vi "FocalSpot.vi"(7 "Racine chemin de sauvegarde":path=path "Z:/Data Gas Experiments/Spring2019/Taches Focales") -> ()   [LabVIEW 2014]
uses:
  <vilib>/addons/PixeLINK/Low Level Functions/ACQUISITION.llb/TDPU-Acquisition-StreamState.ctl
  <vilib>/addons/PixeLINK/Low Level Functions/CAMERA_FEATURES.llb/TDPU-CameraFeatures-FeatureIds.ctl
  <vilib>/addons/PixeLINK/Low Level Functions/CAMERA_FEATURES.llb/TDPU-CameraFeatures-FeatureFlags.ctl
  <vilib>/Analysis/5stat.llb/RMS (DBL).vi
  <vilib>/Analysis/baseanly.llb/Mean (DBL).vi
  <vilib>/Analysis/NI_AALPro.lvlib
  <vilib>/Analysis/NI_AALBase.lvlib
  <vilib>/Utility/file.llb/Write To Spreadsheet File (I64).vi
panel:
  in  "Zoom":bool
  out "rms value":dbl format="%0.2f"
  out "mean":dbl format="%0.2f"
  out "BKG OK":bool
  out "ROI OK":bool
  out "Background":dbl[][](graph)
  in  "Select Background":bool
  out "ROI":dbl[][](graph)
  in  "Select ROI":bool
  in  "Stop Acquisition":bool
  in  "Refresh Exposure":bool
  in  "Transmission":dbl=0.5
  out "Intensity (measured)\nx10^18 W/cm²":dbl=2.0
  out "Div":dbl
  in  "Automatic\nfolder naming":bool=TRUE
  in  "Imager":u32(ring) items=["Low Res Side View"=957000275, "Focal Spot"=953000197, "High Res Side View"=95300230]
  out "?":dbl[][](graph)
  out "?":dbl[][](graph)
  in  "Background  substraction":bool
  out "Intensity (gaussian)\nx10^18 W/cm²":dbl=2.0
  out "Peak power (TW)":dbl=2.0
  out "FWHM y (µm)":dbl=2.0
  out "FWHM x (µm)":dbl=2.0
  in  "Duration FWHM (fs)":dbl=4.5
  in  "Pulse Energy (mJ)":dbl=5.0
  in  "Calibration µm/px":dbl=0.135
  out "Error OUT 2":errorcluster
  out "Error OUT":errorcluster
  in  "Overwrite?":bool
  in  "Snap current Data":bool
  in  "Save Data":bool
  out "Warning":bool
  out "Message":string
  in  "Indice":u32
  in  "Nom du fichier":string="TacheFocale"
  in  "Mode de Sauvegarde":u16(ring)=1 items=["Manuel", "Automatique"]
  out "Focal Spot":dbl[][](graph)
  out "Waiting for Trigger":bool
  in  "Continuous Grab":bool
  in  "Snap Next frame":bool
  out "Camera Handle":u32
  in  "Trigger Type":enum16{"Free Running", "Software", "Hardware"}(ring)
  in  "Trigger Polarity":enum16{"Positive", "Negative"}(ring)
  in  "Refresh Trigger":bool
  in  "Exposure Time":dbl(slide) min=0.0 max=0.0 scale=0.01..10.0
  in  "stop":bool
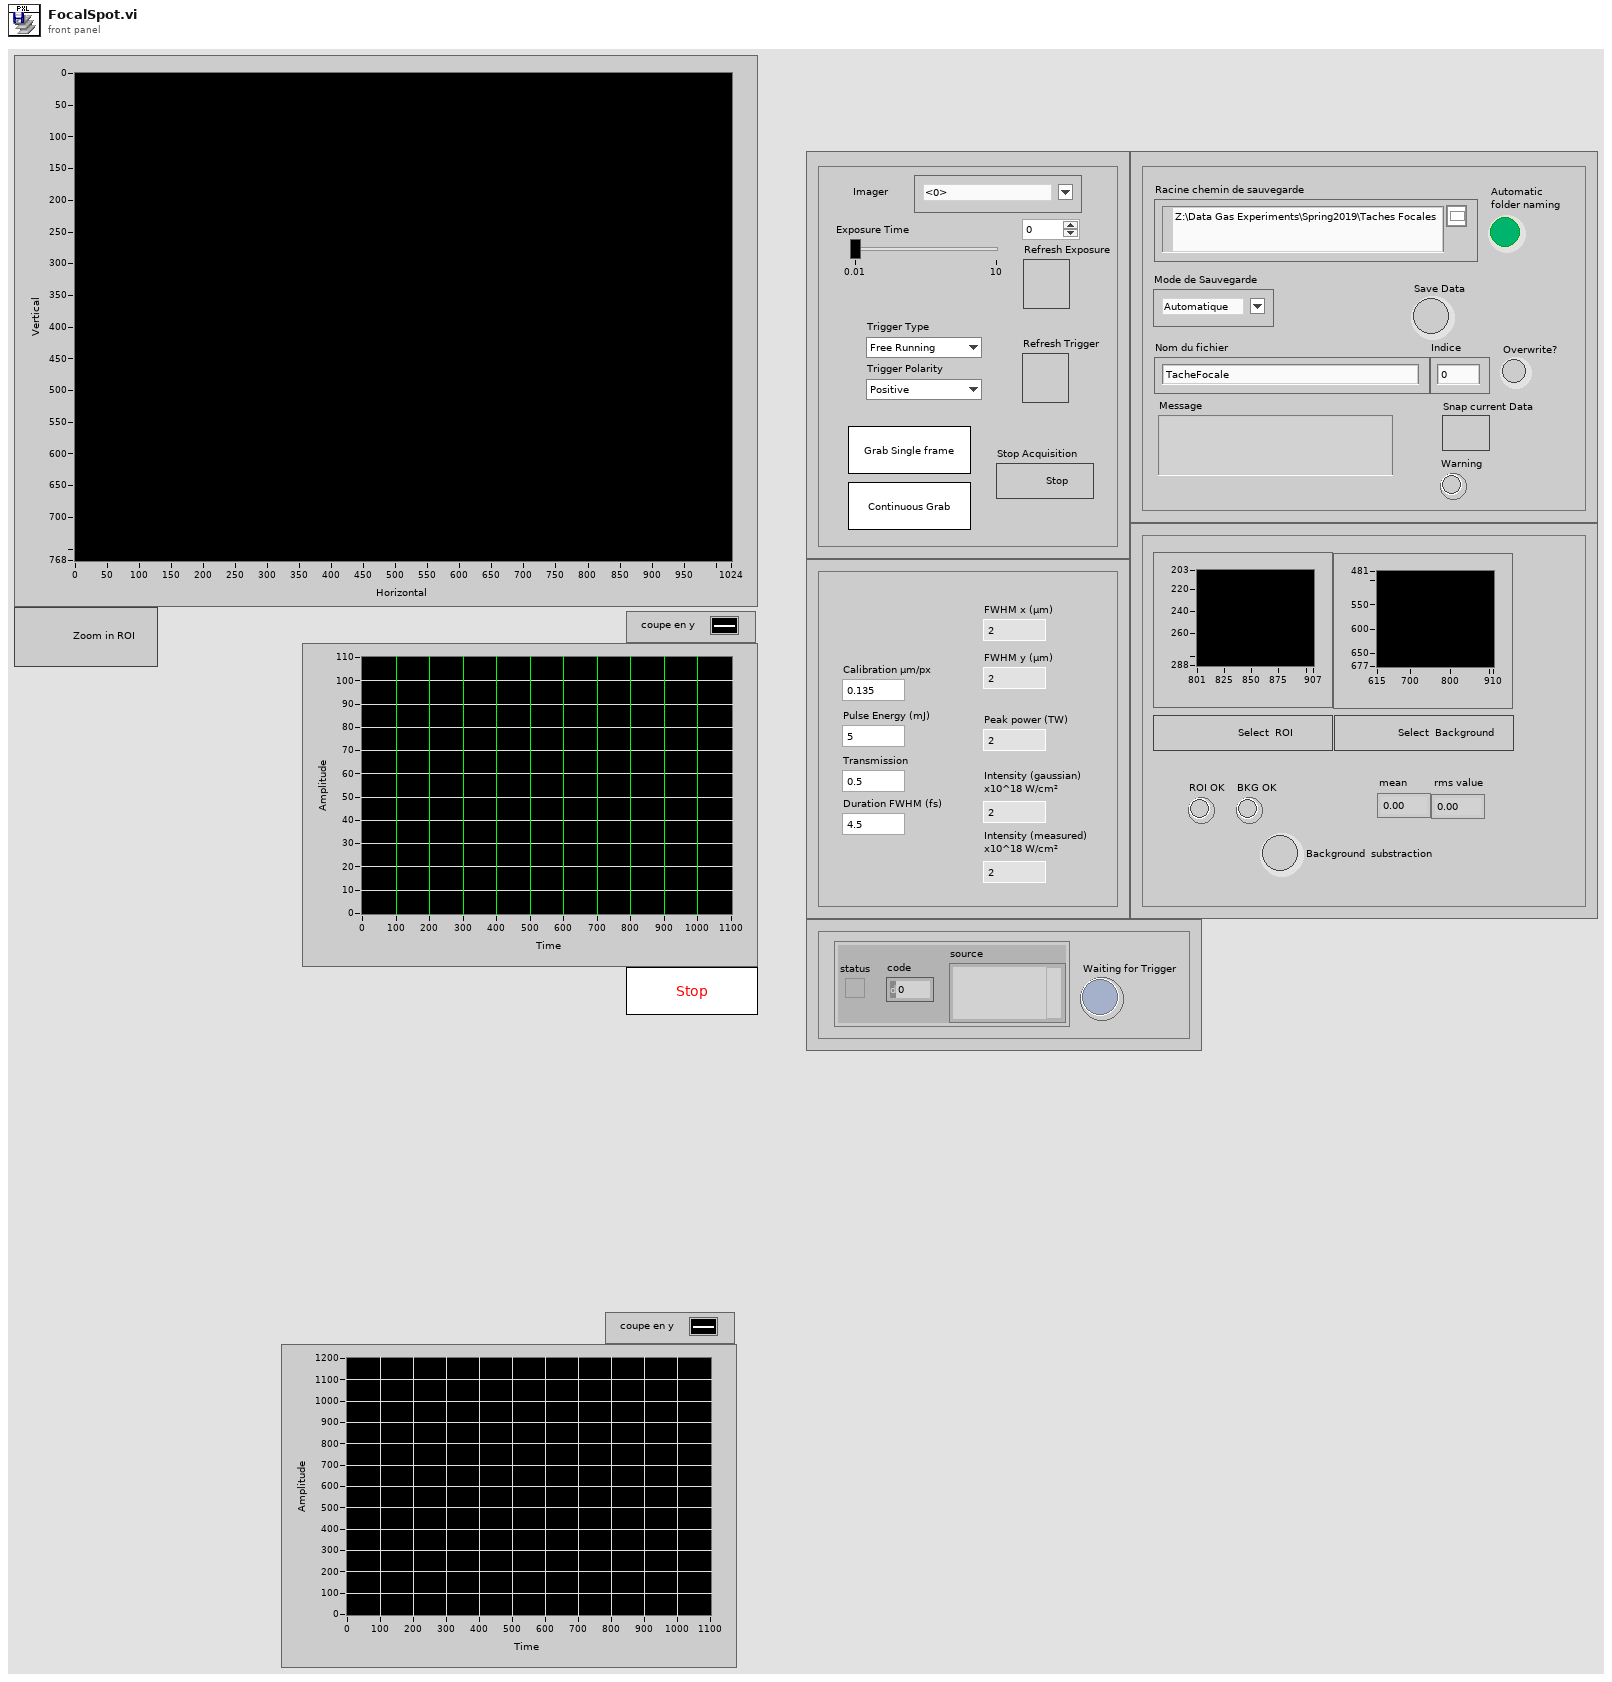
[diagram p1: front panel]
types:
  T1 = typedef "LVStringsAndValuesArrayTypeDef_U32.ctl" = cluster{"String":string, "Value":u32}[]
  T2 = typedef "TDPU-CameraFeatures-FeatureFlags.ctl" = u32
  T3 = typedef "TDPU-CameraFeatures-FeatureIds.ctl" = u32
  T4 = typedef "TDPU-Acquisition-StreamState.ctl" = u32
  T5 = typedef "TDPU-Identification-Camera_Info.ctl" = cluster{"VendorName":string, "ModelName":string, "Description":string, "SerialNumber":string, "FirmwareVersion":string, "FPGAVersion":string, "CameraName":string}
  T6 = typedef "TDPU-Acquisition-Frame_Desc.ctl" = cluster{"uSize":u32, "fFrameTime":dbl, "uFrameNumber":u32, "Brightness":cluster{"fValue":dbl}, "AutoExposure":cluster{"fValue":dbl}, "Sharpness":cluster{"fValue":dbl}, "WhiteBalance":cluster{"fValue":dbl}, "Hue":cluster{"fValue":dbl}, "Saturation":cluster{"fValue":dbl}, "Gamma":cluster{"fValue":dbl}, "Shutter":cluster{"fValue":dbl}, "Gain":cluster{"fValue":dbl}, "Iris":cluster{"fValue":dbl}, "Focus":cluster{"fValue":dbl}, "Temperature":cluster{"fValue":dbl}, "Trigger":cluster{"fMode":dbl, "fType":dbl, "fPolarity":dbl, "fDelay":dbl, "fParameter":dbl}, "Zoom":cluster{"fValue":dbl}, "Pan":cluster{"fValue":dbl}, "Tilt":cluster{"fValue":dbl}, "OpticalFilter":cluster{"fValue":dbl}, "GPIO":cluster{"fMode":dbl[], "fPolarity":dbl[], "fParameter1":dbl[], "fParameter2":dbl[], "fParameter3":dbl[]}, "FrameRate":cluster{"fValue":dbl}, "ROI":cluster{"fLeft":dbl, "fTop":dbl, "fWidth":dbl, "fHeight":dbl}, "Flip":cluster{"fHorizontal":dbl, "fVertical":dbl}, "PixelAddressingValue":cluster{"fValue":dbl}, "PixelFormat":cluster{"fValue":dbl}, "ExtendedShutter":cluster{"fKneePoint":dbl[]}, "AutoROI":cluster{"fLeft":dbl, "fTop":dbl, "fWidth":dbl, "fHeight":dbl}, "WhiteShading":cluster{"fRedGain":dbl, "fGreenGain":dbl, "fBlueGain":dbl}, "Rotate":cluster{"fValue":dbl}, "PixelAddressingMode":cluster{"fValue":dbl}}
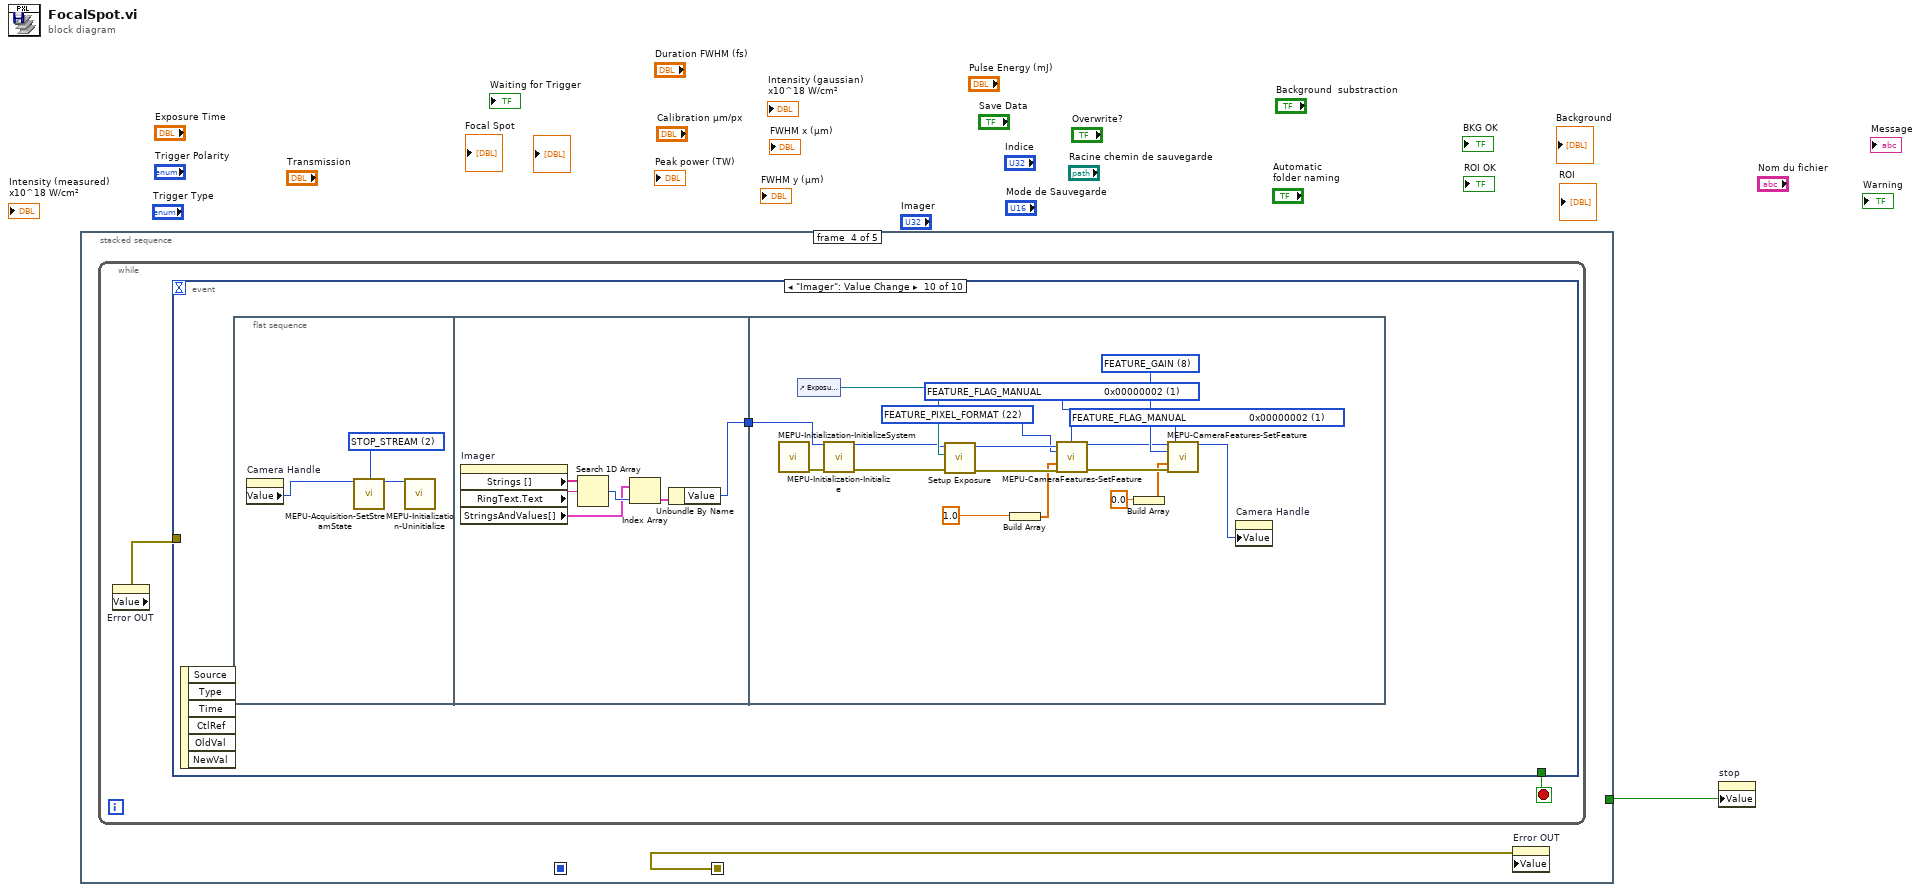
[diagram p0: block diagram]
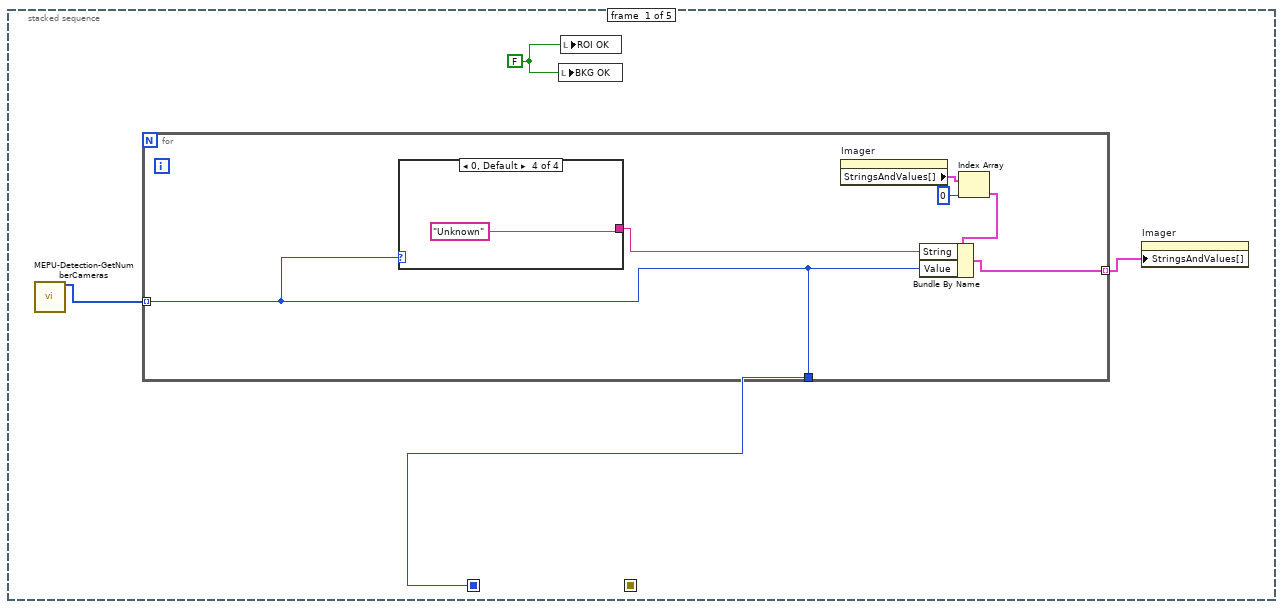
[diagram p2: hidden frame]
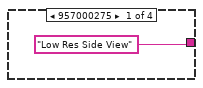
[diagram p3: hidden frame]
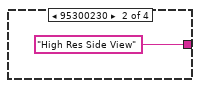
[diagram p4: hidden frame]
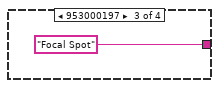
[diagram p5: hidden frame]
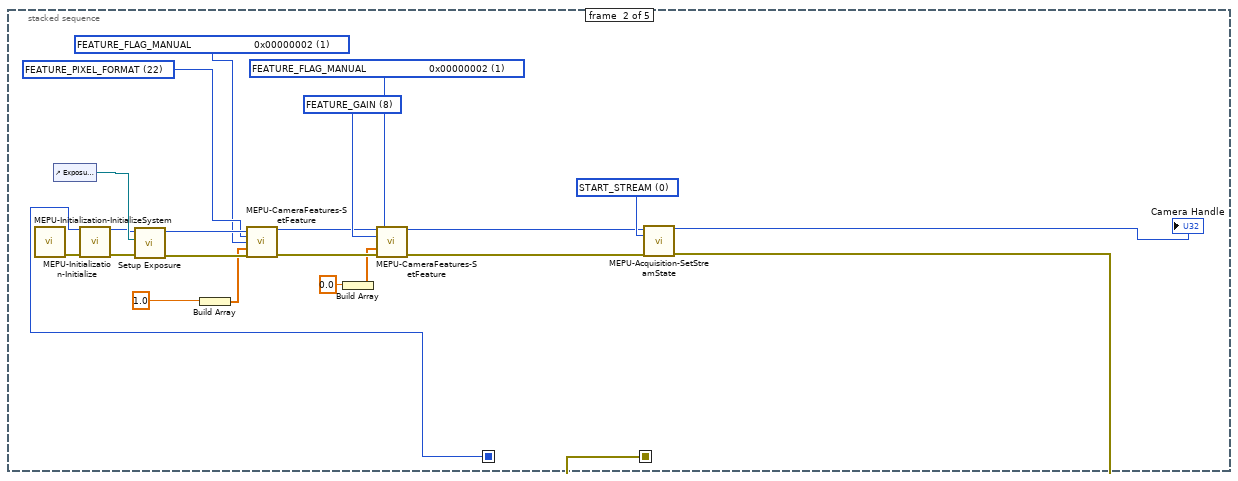
[diagram p6: hidden frame]
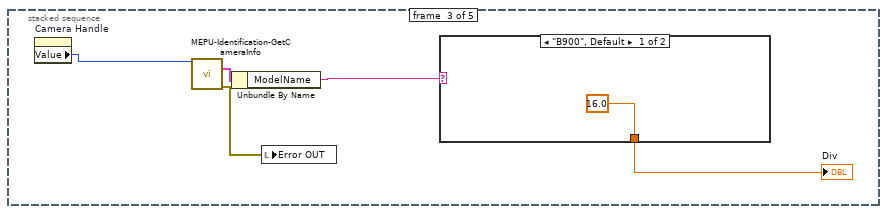
[diagram p7: hidden frame]
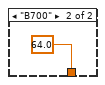
[diagram p8: hidden frame]
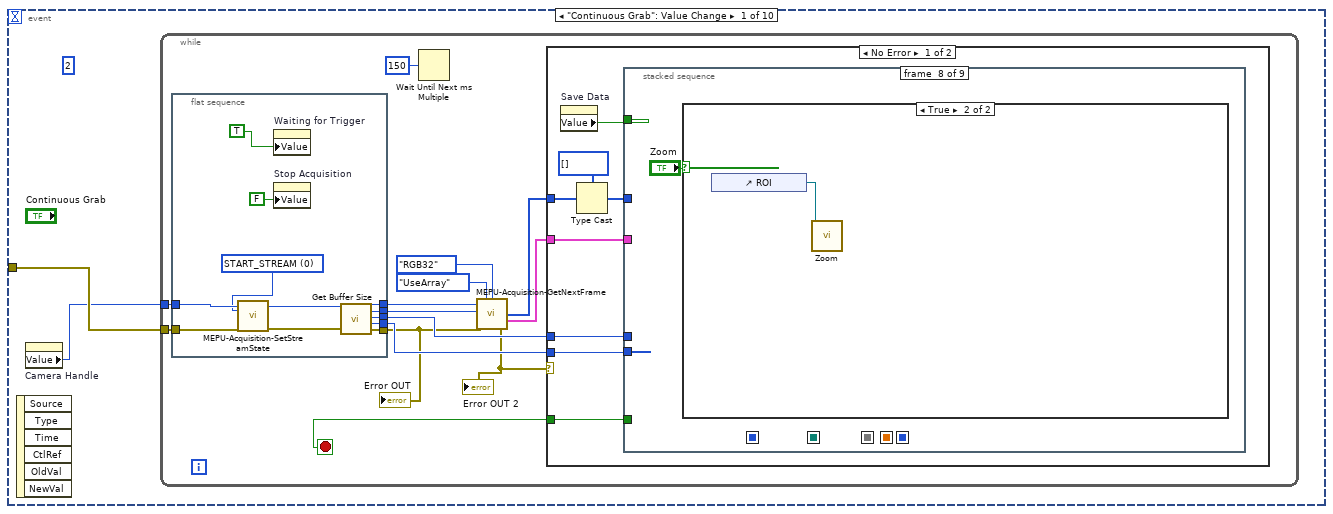
[diagram p9: hidden frame]
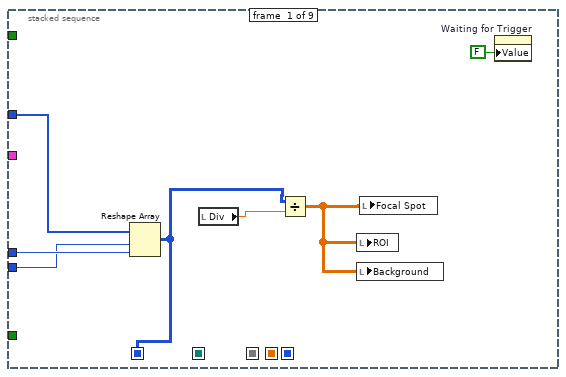
[diagram p10: hidden frame]
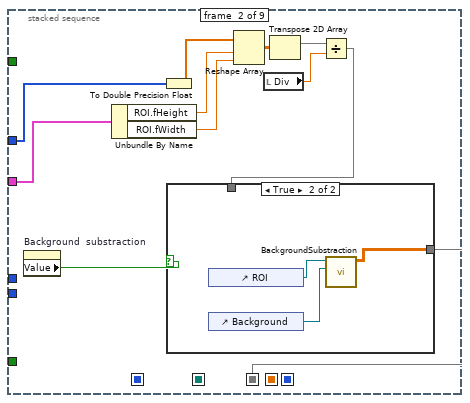
[diagram p11: hidden frame]
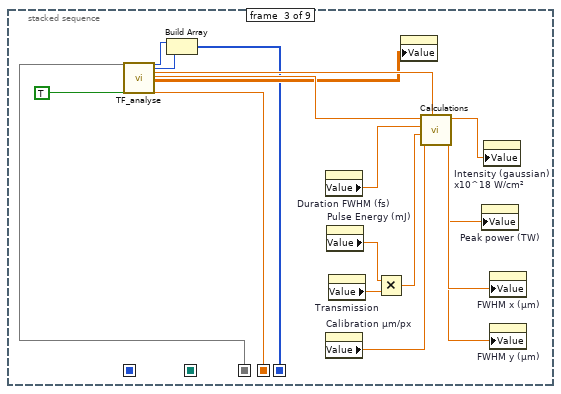
[diagram p13: hidden frame]
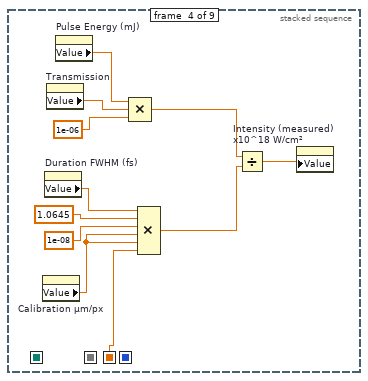
[diagram p14: hidden frame]
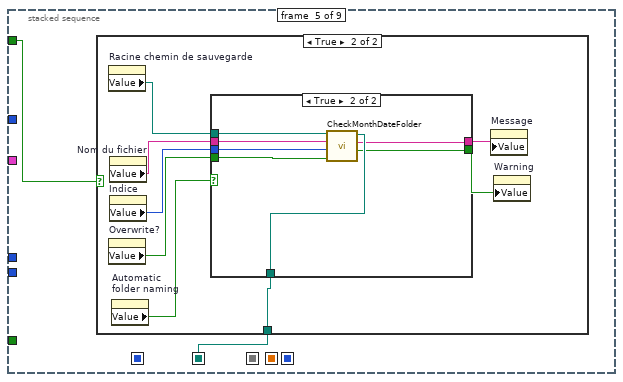
[diagram p15: hidden frame]
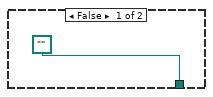
[diagram p16: hidden frame]
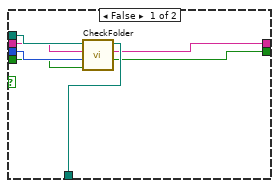
[diagram p17: hidden frame]
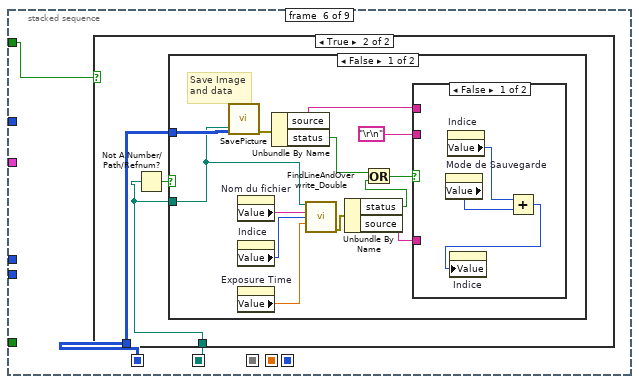
[diagram p18: hidden frame]
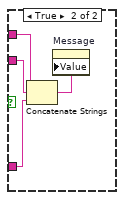
[diagram p20: hidden frame]
diagram:
  n1 = stacked-sequence {
    seq-local: [_ w26 _ _ _] -> [_ _ _ w45 _]
    seq-local: [w3 _ _ _ _] -> [_ w16 _ _ _]
    tunnel: [_ _ _ _ TRUE] -> w1
    frame #0 {
      w2 = FALSE
      n2 = call <vilib>:"MEPU-Detection-GetNumberCameras.vi"() -> ("LV_SerialNumbers OUT"=w5:u32[])  [unwired: 13 in, 2 out]
      n3 = for {
        tunnel: w5 -> [w7] mode=indexing
        tunnel: [w8] -> w4 mode=indexing
        tunnel: [w7] -> w3
        n4 = case shown="0, Default" w7 {
          tunnel: ["Low Res Side View" "High Res Side View" "Focal Spot" "Unknown"] -> w6
          frame 957000275 {
          }
          frame 95300230 {
          }
          frame 953000197 {
          }
          frame 0, Default {
          }
        }
        n5 = property on="Imager" class="Ring (strict)"() -> ("StringsAndValues[]"=w11:T1)  [unwired: 2 in, 2 out]
        n6 = Index Array(array=w11, index=0) -> (element=w9:cluster{"String":string, "Value":u32})
        n7 = Bundle By Name(cluster=w9, "String"=w6, "Value"=w7) -> (w8:cluster{"String":string, "Value":u32})
      }
      n8 = local write "BKG OK"(w2) -> ()
      n9 = local write "ROI OK"(w2) -> ()
      n10 = property on="Imager" class="Ring (strict)"("StringsAndValues[]"=w4) -> ()  [unwired: 2 in, 2 out]
    }
    frame #1 {
      w21 = T2 1 items=["FEATURE_FLAG_PRESENCE                 0x00000001", "FEATURE_FLAG_MANUAL                     0x00000002", "FEATURE_FLAG_AUTO                         0x00000004", "FEATURE_FLAG_ONEPUSH                   0x00000008", "FEATURE_FLAG_OFF                            0x00000010", "FEATURE_FLAG_DESC_SUPPORTED    0x00000020", "FEATURE_FLAG_READ_ONLY               0x00000040"] ("uFlags IN")
      w20 = T3 8 items=["FEATURE_BRIGHTNESS", "FEATURE_EXPOSURE", "FEATURE_SHARPNESS", "FEATURE_WHITE_BAL", "FEATURE_HUE", "FEATURE_SATURATION", "FEATURE_GAMMA", "FEATURE_SHUTTER", "FEATURE_GAIN", "FEATURE_IRIS", "FEATURE_FOCUS", "FEATURE_TEMPERATURE", "FEATURE_TRIGGER", "FEATURE_ZOOM", "FEATURE_PAN", "FEATURE_TILT", "FEATURE_OPT_FILTER", "FEATURE_GPIO", "FEATURE_FRAME_RATE", "FEATURE_ROI", "FEATURE_FLIP", "FEATURE_PIXEL_ADDRESSING", "FEATURE_PIXEL_FORMAT", "FEATURE_EXTENDED_SHUTTER", "FEATURE_AUTO_ROI", "FEATURE_LOOKUP_TABLE", "FEATURE_MEMORY_CHANNEL", "FEATURE_WHITE_SHADING", "FEATURE_ROTATE", "FEATURE_IMAGER_CLK_DIVISOR", "FEATURE_TRIG_WITH_CNTRLD_LIGHT", "FEATURE_MAX_PIXEL_SIZE"] ("uFeatureId IN")
      w29 = T2 1 items=["FEATURE_FLAG_PRESENCE                 0x00000001", "FEATURE_FLAG_MANUAL                     0x00000002", "FEATURE_FLAG_AUTO                         0x00000004", "FEATURE_FLAG_ONEPUSH                   0x00000008", "FEATURE_FLAG_OFF                            0x00000010", "FEATURE_FLAG_DESC_SUPPORTED    0x00000020", "FEATURE_FLAG_READ_ONLY               0x00000040"] ("uFlags IN")
      w30 = T3 22 items=["FEATURE_BRIGHTNESS", "FEATURE_EXPOSURE", "FEATURE_SHARPNESS", "FEATURE_WHITE_BAL", "FEATURE_HUE", "FEATURE_SATURATION", "FEATURE_GAMMA", "FEATURE_SHUTTER", "FEATURE_GAIN", "FEATURE_IRIS", "FEATURE_FOCUS", "FEATURE_TEMPERATURE", "FEATURE_TRIGGER", "FEATURE_ZOOM", "FEATURE_PAN", "FEATURE_TILT", "FEATURE_OPT_FILTER", "FEATURE_GPIO", "FEATURE_FRAME_RATE", "FEATURE_ROI", "FEATURE_FLIP", "FEATURE_PIXEL_ADDRESSING", "FEATURE_PIXEL_FORMAT", "FEATURE_EXTENDED_SHUTTER", "FEATURE_AUTO_ROI", "FEATURE_LOOKUP_TABLE", "FEATURE_MEMORY_CHANNEL", "FEATURE_WHITE_SHADING", "FEATURE_ROTATE", "FEATURE_IMAGER_CLK_DIVISOR", "FEATURE_TRIG_WITH_CNTRLD_LIGHT", "FEATURE_MAX_PIXEL_SIZE"] ("uFeatureId IN")
      w36 = T4 0 items=["START_STREAM", "PAUSE_STREAM", "STOP_STREAM"] ("uStreamState IN")
      n11 = call <vilib>:"MEPU-Initialization-InitializeSystem.vi"() -> ("Error OUT"=w37:errorcluster)  [unwired: 15 in]
      n12 = control-ref of="Exposure Time"() -> (w35:refnum<vi>)
      n13 = call <vilib>:"MEPU-Initialization-Initialize.vi"("uSerialNumber IN"=w16, "Error IN"=w37) -> ("phCamera OUT"=w34:u32, "Error OUT"=w33:errorcluster)  [unwired: 11 in, 1 out]
      n14 = call "Setup Exposure.vi"("Error IN"=w33, "Shutter"=w35, "hCamera IN"=w34) -> ("Error OUT"=w32:errorcluster, "phCamera OUT"=w31:u32)  [unwired: 7 in]
      n15 = Build Array(1.0) -> (w27:dbl[])
      n16 = call <vilib>:"MEPU-CameraFeatures-SetFeature.vi"("hCamera IN"=w31, "uFeatureId IN"=w30, "uFlags IN"=w29, "pParms IN"=w27, "Error IN"=w32) -> ("hCamera OUT"=w19:u32, "Error OUT"=w24:errorcluster)  [unwired: 8 in, 1 out]
      n17 = Build Array(0.0) -> (w22:dbl[])
      n18 = call <vilib>:"MEPU-CameraFeatures-SetFeature.vi"("hCamera IN"=w19, "uFeatureId IN"=w20, "uFlags IN"=w21, "pParms IN"=w22, "Error IN"=w24) -> ("hCamera OUT"=w18:u32, "Error OUT"=w17:errorcluster)  [unwired: 8 in, 1 out]
      n19 = call <vilib>:"MEPU-Acquisition-SetStreamState.vi"("hCamera IN"=w18, "uStreamState IN"=w36, "Error IN"=w17) -> ("hCamera OUT"=→"Camera Handle":u32, "Error OUT"=w26:errorcluster)  [unwired: 11 in]
    }
    frame #2 {
      n20 = property on="Camera Handle" class="DigNum (strict)"() -> ("Value"=w41:u32)  [unwired: 2 in, 2 out]
      n21 = call <vilib>:"MEPU-Identification-GetCameraInfo.vi"("hCamera IN"=w41) -> ("pLVCameraInfo OUT"=w42:T5, "Error OUT"=w38:errorcluster)  [unwired: 12 in, 1 out]
      n22 = Unbundle By Name(w42) -> ("ModelName"=w40:string)
      n23 = local write "Error OUT"(w38) -> ()
      n24 = case shown="\"B900\", Default" w40 {
        tunnel: [16.0 64.0] -> w39
        frame "B900", Default {
        }
        frame "B700" {
        }
      }
      "Div" <- w39
    }
    frame #3 {
      n25 = while {
        stop <- w47 stop-if-true
        n26 = property on="Error OUT" class="Clust (strict)"() -> ("Value"=w46:errorcluster)  [unwired: 2 in, 2 out]
        n27 = event shown="[9] \"Imager\": Value Change" {
          selector: _ -> [_ _ _ _ _ _ _ _ _ _]
          dyn-events: _ -> [_ _ _ _ _ _ _ _ _ _]
          timeout: _ -> [_ _ _ _ _ _ _ _ _ _]
          tunnel: w46 -> [w49 _ _ _ _ _ w237 w256 _ _]
          tunnel: [_ _ _ _ _ TRUE _ _ _ _] -> w47
          event "Continuous Grab": Value Change {
            (unwired) i64 2 ("Period")
            n28 = event-data() -> ()  [unwired: 1 in, 6 out]
            n29 = property on="Camera Handle" class="DigNum (strict)"() -> ("Value"=w48:u32)  [unwired: 2 in, 2 out]
            n30 = while {
              tunnel: w48 -> [w63]
              tunnel: w49 -> [w57]
              stop <- w51 stop-if-true
              n31 = flat-sequence {
                tunnel: w63 -> [w186]
                tunnel: [w195] -> w62
                tunnel: [w194] -> w61
                tunnel: [w193] -> w54
                tunnel: w57 -> [w189]
                tunnel: [w192] -> w56
                tunnel: [w191] -> w55
                frame #0 {
                  w185 = T4 0 items=["START_STREAM", "PAUSE_STREAM", "STOP_STREAM"] ("uStreamState IN")
                  n32 = call <vilib>:"MEPU-Acquisition-SetStreamState.vi"("hCamera IN"=w186, "uStreamState IN"=w185, "Error IN"=w189) -> ("hCamera OUT"=w187:u32, "Error OUT"=w188:errorcluster)  [unwired: 11 in]
                  n33 = property on="Waiting for Trigger" class="Bool (strict)"("Value"=TRUE ("Waiting for Trigger")) -> ()  [unwired: 2 in, 2 out]
                  n34 = property on="Stop Acquisition" class="Bool (strict)"("Value"=FALSE ("Stop Acquisition")) -> ()  [unwired: 2 in, 2 out]
                  n35 = call "Get Buffer Size.vi"("phCamera IN"=w187, "Error IN"=w188) -> ("phCamera OUT"=w195:u32, "uBufferSize OUT"=w194:u32, "uWidth OUT"=w192:u32, "uHeight OUT"=w191:u32, "Error OUT"=w193:errorcluster)  [unwired: 8 in, 1 out]
                }
              }
              n36 = Wait Until Next ms Multiple(millisecond multiple=u32 150) -> ()  [unwired: 1 out]
              n37 = call <vilib>:"MEPU-Acquisition-GetNextFrame.vi"("hCamera IN"=w62, "Mode IN"=enum16{"UseArray", "UsePointer"}."UseArray", "OutputMode IN"=enum16{"Default", "RGB24", "RGB32"}."RGB32", "uBufferSize IN"=w61, "Error IN"=w54) -> ("Data OUT"=w58:u8[], "pDescriptor"=w52:T6, "Error OUT"=w53:errorcluster)  [unwired: 6 in, 2 out]
              "Error OUT 2" <- w53
              n38 = case shown="No Error" w53 {
                tunnel: w58 -> [w71 _]
                tunnel: w56 -> [w68 _]
                tunnel: w55 -> [w67 _]
                tunnel: w52 -> [w65 _]
                tunnel: [w64 w183] -> w51
                frame No Error {
                  n39 = property on="Save Data" class="Bool (strict)"() -> ("Value"=w66:bool)  [unwired: 2 in, 2 out]
                  n40 = Type Cast(type=u16[] [] ("Data OUT"), x=w71) -> (*(type *) &x=w69:u16[])
                  n41 = stacked-sequence {
                    seq-local: [_ _ _ _ w124 _ _ _ _] -> [_ _ _ _ _ w150 _ _ _]
                    seq-local: [_ w79 _ _ _ _ _ _ _] -> [_ _ w110 _ _ _ _ _ _]
                    seq-local: [w74 _ _ _ _ _ _ _ _] -> [_ _ _ _ _ w148 _ _ _]
                    seq-local: [_ _ w100 _ _ _ _ _ _] -> [_ _ _ w112 _ _ _ _ _]
                    seq-local: [_ _ w94 _ _ _ _ _ _] -> [_ _ _ _ _ _ w174 _ _]
                    tunnel: w69 -> [w78 w86 _ _ _ _ _ _ _]
                    tunnel: w68 -> [w77 _ _ _ _ _ _ _ _]
                    tunnel: w67 -> [w76 _ _ _ _ _ _ _ _]
                    tunnel: w66 -> [_ _ _ _ w123 w149 _ _ _]
                    tunnel: w65 -> [_ w89 _ _ _ _ _ _ _]
                    tunnel: [_ _ _ _ _ _ _ _ "Stop Acquisition"] -> w64
                    frame #0 {
                      n42 = Reshape Array(w78, w76, w77) -> (w74:u16[][])
                      n43 = local read "Div"() -> (w73:dbl)
                      n44 = Divide(x=w74, y=w73) -> (x/y=w72:dbl[][])
                      n45 = local write "ROI"(w72) -> ()
                      n46 = local write "Background"(w72) -> ()
                      n47 = local write "Focal Spot"(w72) -> ()
                      n48 = property on="Waiting for Trigger" class="Bool (strict)"("Value"=FALSE ("Waiting for Trigger")) -> ()  [unwired: 2 in, 2 out]
                    }
                    frame #1 {
                      n49 = property on="Background  substraction" class="Bool (strict)"() -> ("Value"=w83:bool)  [unwired: 2 in, 2 out]
                      n50 = Unbundle By Name(w89) -> ("ROI.fHeight"=w88:dbl, "ROI.fWidth"=w87:dbl)
                      n51 = To Double Precision Float(number=w86) -> (double precision float=w84:dbl[])
                      n52 = Reshape Array(w84, w88, w87) -> (w85:dbl[][])
                      n53 = local read "Div"() -> (w81:dbl)
                      n54 = Transpose 2D Array(2D array=w85) -> (transposed array=w82:dbl[][])
                      n55 = Divide(x=w82, y=w81) -> (x/y=w80:dbl[][])
                      n56 = case shown="True" w83 {
                        tunnel: w80 -> [w90 _]
                        tunnel: [w90 w91] -> w79
                        frame False {
                        }
                        frame True {
                          n57 = control-ref of="ROI"() -> (w93:refnum<vi>)
                          n58 = control-ref of="Background"() -> (w92:refnum<vi>)
                          n59 = call "BackgroundSubstraction.vi"("Background Refnum"=w92, "ROI Refnum"=w93) -> ("Background Sub ROI"=w91:dbl[][])  [unwired: 9 in]
                        }
                      }
                    }
                    frame #2 {
                      n60 = call "TF_analyse.vi"("image 2D"=w110, "FLUENCE calculation"=TRUE) -> ("position max en x"=w96:i32, "position max en y"=w95:i32, "FWHM en x"=w106:dbl, "FWHM en y"=w107:dbl, "coupes x & y"=w101:dbl[][], "intégration totale"=w100:dbl)  [unwired: 19 in, 1 out]
                      n61 = Build Array(w96, w95) -> (w94:i32[])
                      n62 = property on="Duration FWHM (fs)" class="DigNum (strict)"() -> ("Value"=w108:dbl)  [unwired: 2 in, 2 out]
                      n63 = property on="Calibration µm/px" class="DigNum (strict)"() -> ("Value"=w109:dbl)  [unwired: 2 in, 2 out]
                      n64 = property on="Pulse Energy (mJ)" class="DigNum (strict)"() -> ("Value"=w98:dbl)  [unwired: 2 in, 2 out]
                      n65 = property on="Transmission" class="DigNum (strict)"() -> ("Value"=w99:dbl)  [unwired: 2 in, 2 out]
                      n66 = Multiply(x=w98, y=w99) -> (x*y=w97:dbl)
                      n67 = property class="WFGraph (strict)"("Value"=w101) -> ()  [unwired: 2 in, 2 out]
                      n68 = call "Calculations.vi"("FWHM x (px)"=w106, "Calibration µm/px"=w109, "Energy in 1 Pulse (mJ)"=w97, "Pulse Duration (fs)"=w108, "FWHM y (px)"=w107) -> ("FWHM y (µm)"=w104:dbl, "FWHM x (µm)"=w105:dbl, "Peak Power (TW)"=w103:dbl, "Integral of Perfect Gaussian (x10^18 W/cm²)"=w102:dbl)  [unwired: 3 in]
                      n69 = property on="Peak power (TW)" class="DigNum (strict)"("Value"=w103) -> ()  [unwired: 2 in, 2 out]
                      n70 = property on="Intensity (gaussian)\nx10^18 W/cm²" class="DigNum (strict)"("Value"=w102) -> ()  [unwired: 2 in, 2 out]
                      n71 = property on="FWHM x (µm)" class="DigNum (strict)"("Value"=w105) -> ()  [unwired: 2 in, 2 out]
                      n72 = property on="FWHM y (µm)" class="DigNum (strict)"("Value"=w104) -> ()  [unwired: 2 in, 2 out]
                    }
                    frame #3 {
                      n73 = property on="Calibration µm/px" class="DigNum (strict)"() -> ("Value"=w116:dbl)  [unwired: 2 in, 2 out]
                      n74 = property on="Duration FWHM (fs)" class="DigNum (strict)"() -> ("Value"=w119:dbl)  [unwired: 2 in, 2 out]
                      n75 = property on="Transmission" class="DigNum (strict)"() -> ("Value"=w121:dbl)  [unwired: 2 in, 2 out]
                      n76 = property on="Pulse Energy (mJ)" class="DigNum (strict)"() -> ("Value"=w122:dbl)  [unwired: 2 in, 2 out]
                      n77 = Compound Arithmetic op=MULTIPLY(w122, w121, 1e-06 ("Transmission")) -> (w115:dbl)
                      n78 = Compound Arithmetic op=MULTIPLY(w119, 1.0645 ("Transmission"), 1e-08 ("Transmission"), w116, w116, w112) -> (w114:dbl)
                      n79 = Divide(x=w115, y=w114) -> (x/y=w113:dbl)
                      n80 = property on="Intensity (measured)\nx10^18 W/cm²" class="DigNum (strict)"("Value"=w113) -> ()  [unwired: 2 in, 2 out]
                    }
                    frame #4 {
                      n81 = case shown="True" w123 {
                        tunnel: [path "" ("File Path") w129] -> w124
                        frame False {
                        }
                        frame True {
                          n82 = property on="Racine chemin de sauvegarde" class="Path"() -> ("Value"=w130:path)  [unwired: 2 in, 2 out]
                          n83 = property on="Overwrite?" class="Bool (strict)"() -> ("Value"=w133:bool)  [unwired: 2 in, 2 out]
                          n84 = property on="Nom du fichier" class="Str"() -> ("Value"=w131:string)  [unwired: 2 in, 2 out]
                          n85 = property on="Indice" class="DigNum (strict)"() -> ("Value"=w132:u32)  [unwired: 2 in, 2 out]
                          n86 = property on="Automatic\nfolder naming" class="Bool (strict)"() -> ("Value"=w126:bool)  [unwired: 2 in, 2 out]
                          n87 = case shown="True" w126 {
                            tunnel: w133 -> [w137 w147]
                            tunnel: w132 -> [w138 w146]
                            tunnel: w131 -> [w139 w145]
                            tunnel: w130 -> [w140 w144]
                            tunnel: [w136 w143] -> w129
                            tunnel: [w135 w142] -> w128
                            tunnel: [w134 w141] -> w127
                            frame False {
                              n88 = call "CheckFolder.vi"("Overwrite?"=w137, "Index"=w138, "File Name"=w139, "Folder Path Control"=w140) -> ("Warning"=w134:bool, "Message"=w135:string, "File Path"=w136:path)  [unwired: 5 in]
                            }
                            frame True {
                              n89 = call "CheckMonthDateFolder.vi"("Overwrite?"=w147, "Index"=w146, "File Name"=w145, "Folder Path Control"=w144) -> ("Warning"=w141:bool, "Message"=w142:string, "File Path"=w143:path)  [unwired: 5 in]
                            }
                          }
                          n90 = property on="Message" class="Str"("Value"=w128) -> ()  [unwired: 2 in, 2 out]
                          n91 = property on="Warning" class="Bool (strict)"("Value"=w127) -> ()  [unwired: 2 in, 2 out]
                        }
                      }
                    }
                    frame #5 {
                      n92 = case shown="True" w149 {
                        tunnel: w150 -> [_ w152]
                        tunnel: w148 -> [_ w151]
                        frame False {
                        }
                        frame True {
                          n93 = Not A Number/Path/Refnum?(number/path/refnum=w152) -> (NaN/Path/Refnum?=w153:bool)
                          n94 = case shown="False" w153 {
                            tunnel: w152 -> [w156 _]
                            tunnel: w151 -> [w159 _]
                            frame False {
                              # "Save Image\nand data"
                              n95 = call "SavePicture.vi"("File Path"=w156, "Image Pixels (U16)"=w159) -> ("error out"=w165:errorcluster)  [unwired: 9 in]
                              n96 = property on="Nom du fichier" class="Str"() -> ("Value"=w157:string)  [unwired: 2 in, 2 out]
                              n97 = property on="Indice" class="DigNum (strict)"() -> ("Value"=w155:u32)  [unwired: 2 in, 2 out]
                              n98 = property on="Exposure Time" class="Slide (strict)"() -> ("Value"=w154:dbl)  [unwired: 2 in, 2 out]
                              n99 = Unbundle By Name(w165) -> ("source"=w162:string, "status"=w163:bool)
                              n100 = call "FindLineAndOverwrite_Double.vi"("Exposure path"=w156, "Name"=w157, "Index"=w155, "Exposure"=w154) -> ("error out"=w158:errorcluster)  [unwired: 11 in]
                              n101 = Unbundle By Name(w158) -> ("status"=w164:bool, "source"=w166:string)
                              n102 = Or(x=w163, y=w164) -> (x .or. y?=w161:bool)
                              n103 = case shown="False" w161 {
                                tunnel: w166 -> [_ w170]
                                tunnel: w162 -> [_ w173]
                                tunnel: "\r\n" -> [_ w171]
                                frame False {
                                n104 = property on="Mode de Sauvegarde" class="Ring (strict)"() -> ("Value"=w168:u16)  [unwired: 2 in, 2 out]
                                n105 = property on="Indice" class="DigNum (strict)"() -> ("Value"=w169:u32)  [unwired: 2 in, 2 out]
                                n106 = Add(x=w169, y=w168) -> (x+y=w167:u32)
                                n107 = property on="Indice" class="DigNum (strict)"("Value"=w167) -> ()  [unwired: 2 in, 2 out]
                                }
                                frame True {
                                n108 = Concatenate Strings(w173, w171, w170) -> (w172:string)
                                n109 = property on="Message" class="Str"("Value"=w172) -> ()  [unwired: 2 in, 2 out]
                                }
                              }
                            }
                            frame True {
                            }
                          }
                        }
                      }
                    }
                    frame #6 {
                      n110 = disable-structure shown="Disabled" {
                        disable-tunnel: w174 -> [w175 _]
                        frame Disabled {
                          n111 = Build Path(base path=path "Z:/Data Gas Experiments/Spring2017/Mechanical stability/SalleNoire_to_SalleOrange", name or relative path="xyJitter17h40.dat") -> (appended path=w177:path)
                          n112 = call-poly <vilib>:"Write To Spreadsheet File.vi"("append to file? (new file:F)"=TRUE, "1D data"=w175, "file path (dialog if empty)"=w177) -> ()  [unwired: 5 in, 1 out]
                        }
                        frame Enabled {
                        }
                      }
                    }
                    frame #7 {
                      n113 = case shown="True" "Zoom" {
                        frame False {
                        }
                        frame True {
                          n114 = control-ref of="ROI"() -> (w181:refnum<vi>)
                          n115 = call "Zoom.vi"("IntGraph Refnum"=w181) -> ()  [unwired: 11 in]
                        }
                      }
                    }
                    frame #8 {
                    }
                  }
                }
                frame Error {
                  n116 = property on="Stop Acquisition" class="Bool (strict)"() -> ("Value"=w183:bool)  [unwired: 2 in, 2 out]
                }
              }
              "Error OUT" <- w54
            }
          }
          event "Select ROI": Value Change {
            # "Evaluate Bounds of ROI"
            n117 = event-data() -> ()  [unwired: 1 in, 6 out]
            n118 = control-ref of="Focal Spot"() -> (w198:refnum<vi>)
            n119 = control-ref of="ROI"() -> (w196:refnum<vi>)
            n120 = call "SmartBackground.vi"("ROI"=w196, "Input Graph"=w198) -> ()  [unwired: 10 in]
            n121 = call "Zoom.vi"("IntGraph Refnum"=w196) -> ()  [unwired: 11 in]
            n122 = local write "ROI OK"(TRUE ("BKG OK")) -> ()
          }
          event "Select Background": Value Change {
            # "Evaluate Bounds of Background"
            n123 = event-data() -> ()  [unwired: 1 in, 6 out]
            n124 = flat-sequence {
              tunnel: [w214] -> w211
              tunnel: w211 -> [w220]
              tunnel: [w219] -> w210
              tunnel: [w218] -> w208
              tunnel: [w217] -> w209
              tunnel: [w216] -> w206
              frame #0 {
                n125 = control-ref of="Background"() -> (w214:refnum<vi>)
                n126 = control-ref of="Focal Spot"() -> (w215:refnum<vi>)
                n127 = call "SmartBackground.vi"("ROI"=w214, "Input Graph"=w215) -> ()  [unwired: 10 in]
              }
              frame #1 {
                n128 = property on="Property Node" class="IntGraph (strict)"(reference=w220) -> ("XScale.Maximum"=w219:dbl, "XScale.Minimum"=w218:dbl, "YScale.Maximum"=w217:dbl, "YScale.Minimum"=w216:dbl)  [unwired: 1 in, 2 out]
              }
            }
            n129 = local read "Focal Spot"() -> (w212:dbl[][])
            n130 = Subtract(x=w209, y=w206) -> (x-y=w205:dbl)
            n131 = Subtract(x=w210, y=w208) -> (x-y=w207:dbl)
            n132 = Array Subset(array=w212, index (row)=w208, length (row)=w207, index (col)=w206, length (col)=w205) -> (w204:dbl[][])
            n133 = local write "BKG OK"(TRUE ("BKG OK")) -> ()
            n134 = Array Size(array=w204) -> (size(s)=w201:i32[])
            n135 = Multiply Array Elements(1:w201) -> (0:w202:i32)
            n136 = Reshape Array(w204, w202) -> (w203:dbl[])
            n137 = call-poly <vilib>:"RMS.vi"("X"=w203) -> ("rms value"=→"rms value":dbl)  [unwired: 1 out]
            n138 = call-poly <vilib>:"Mean.vi"("X"=w203) -> ("mean"=→"mean":dbl)  [unwired: 1 out]
          }
          event "Trigger Polarity", "Trigger Type": Value Change {
            n139 = event-data() -> ()  [unwired: 1 in, 6 out]
            n140 = property on="Refresh Trigger" class="Bool"("Blinking"=TRUE) -> ()  [unwired: 2 in, 2 out]
          }
          event "Refresh Exposure": Value Change {
            w225 = T2 1 items=["FEATURE_FLAG_PRESENCE                 0x00000001", "FEATURE_FLAG_MANUAL                     0x00000002", "FEATURE_FLAG_AUTO                         0x00000004", "FEATURE_FLAG_ONEPUSH                   0x00000008", "FEATURE_FLAG_OFF                            0x00000010", "FEATURE_FLAG_DESC_SUPPORTED    0x00000020", "FEATURE_FLAG_READ_ONLY               0x00000040"] ("uFlags IN")
            w226 = T3 7 items=["FEATURE_BRIGHTNESS", "FEATURE_EXPOSURE", "FEATURE_SHARPNESS", "FEATURE_WHITE_BAL", "FEATURE_HUE", "FEATURE_SATURATION", "FEATURE_GAMMA", "FEATURE_SHUTTER", "FEATURE_GAIN", "FEATURE_IRIS", "FEATURE_FOCUS", "FEATURE_TEMPERATURE", "FEATURE_TRIGGER", "FEATURE_ZOOM", "FEATURE_PAN", "FEATURE_TILT", "FEATURE_OPT_FILTER", "FEATURE_GPIO", "FEATURE_FRAME_RATE", "FEATURE_ROI", "FEATURE_FLIP", "FEATURE_PIXEL_ADDRESSING", "FEATURE_PIXEL_FORMAT", "FEATURE_EXTENDED_SHUTTER", "FEATURE_AUTO_ROI", "FEATURE_LOOKUP_TABLE", "FEATURE_MEMORY_CHANNEL", "FEATURE_WHITE_SHADING", "FEATURE_ROTATE", "FEATURE_IMAGER_CLK_DIVISOR", "FEATURE_TRIG_WITH_CNTRLD_LIGHT", "FEATURE_MAX_PIXEL_SIZE"] ("uFeatureId IN")
            n141 = event-data() -> ()  [unwired: 1 in, 6 out]
            n142 = property on="Camera Handle" class="DigNum (strict)"() -> ("Value"=w222:u32)  [unwired: 2 in, 2 out]
            n143 = property on="Exposure Time" class="Slide (strict)"() -> ("Value"=w224:dbl)  [unwired: 2 in, 2 out]
            n144 = Build Array(w224) -> (w223:dbl[])
            n145 = call <vilib>:"MEPU-CameraFeatures-SetFeature.vi"("hCamera IN"=w222, "uFeatureId IN"=w226, "uFlags IN"=w225, "pParms IN"=w223) -> ()  [unwired: 1 in, 11 out]
          }
          event "stop": Value Change {
            n146 = event-data() -> ()  [unwired: 1 in, 6 out]
            n147 = property on="Refresh Trigger" class="Bool"("Blinking"=FALSE) -> ()  [unwired: 2 in, 2 out]
          }
          event "Refresh Trigger": Value Change {
            w231 = T4 2 items=["START_STREAM", "PAUSE_STREAM", "STOP_STREAM"] ("uStreamState IN")
            w232 = T4 0 items=["START_STREAM", "PAUSE_STREAM", "STOP_STREAM"] ("uStreamState IN")
            w246 = T2 1 items=["FEATURE_FLAG_PRESENCE                 0x00000001", "FEATURE_FLAG_MANUAL                     0x00000002", "FEATURE_FLAG_AUTO                         0x00000004", "FEATURE_FLAG_ONEPUSH                   0x00000008", "FEATURE_FLAG_OFF                            0x00000010", "FEATURE_FLAG_DESC_SUPPORTED    0x00000020", "FEATURE_FLAG_READ_ONLY               0x00000040"] ("uFlags IN")
            w247 = T3 12 items=["FEATURE_BRIGHTNESS", "FEATURE_EXPOSURE", "FEATURE_SHARPNESS", "FEATURE_WHITE_BAL", "FEATURE_HUE", "FEATURE_SATURATION", "FEATURE_GAMMA", "FEATURE_SHUTTER", "FEATURE_GAIN", "FEATURE_IRIS", "FEATURE_FOCUS", "FEATURE_TEMPERATURE", "FEATURE_TRIGGER", "FEATURE_ZOOM", "FEATURE_PAN", "FEATURE_TILT", "FEATURE_OPT_FILTER", "FEATURE_GPIO", "FEATURE_FRAME_RATE", "FEATURE_ROI", "FEATURE_FLIP", "FEATURE_PIXEL_ADDRESSING", "FEATURE_PIXEL_FORMAT", "FEATURE_EXTENDED_SHUTTER", "FEATURE_AUTO_ROI", "FEATURE_LOOKUP_TABLE", "FEATURE_MEMORY_CHANNEL", "FEATURE_WHITE_SHADING", "FEATURE_ROTATE", "FEATURE_IMAGER_CLK_DIVISOR", "FEATURE_TRIG_WITH_CNTRLD_LIGHT", "FEATURE_MAX_PIXEL_SIZE"] ("uFeatureId IN")
            n148 = event-data() -> ()  [unwired: 1 in, 6 out]
            n149 = property on="Camera Handle" class="DigNum (strict)"() -> ("Value"=w229:u32)  [unwired: 2 in, 2 out]
            n150 = property on="Refresh Trigger" class="Bool"("Blinking"=FALSE) -> ()  [unwired: 2 in, 2 out]
            n151 = property on="Trigger Polarity" class="Enum (strict)"() -> ("Value"=w242:enum16{"Positive", "Negative"})  [unwired: 2 in, 2 out]
            n152 = property on="Trigger Type" class="Enum (strict)"() -> ("Value"=w244:enum16{"Free Running", "Software", "Hardware"})  [unwired: 2 in, 2 out]
            n153 = To Double Precision Float(number=w242) -> (double precision float=w241:dbl)
            n154 = To Double Precision Float(number=w244) -> (double precision float=w243:dbl)
            n155 = Build Array(0.0 ("element"), w243, w241, 0.0 ("element"), 0.0 ("element")) -> (w238:dbl[])
            n156 = call <vilib>:"MEPU-Acquisition-SetStreamState.vi"("hCamera IN"=w229, "uStreamState IN"=w231, "Error IN"=w237) -> ("hCamera OUT"=w236:u32, "Error OUT"=w235:errorcluster)  [unwired: 11 in]
            n157 = call <vilib>:"MEPU-CameraFeatures-SetFeature.vi"("hCamera IN"=w236, "uFeatureId IN"=w247, "uFlags IN"=w246, "pParms IN"=w238, "Error IN"=w235) -> ("hCamera OUT"=w233:u32, "Error OUT"=w234:errorcluster)  [unwired: 9 out]
            n158 = call <vilib>:"MEPU-Acquisition-SetStreamState.vi"("hCamera IN"=w233, "uStreamState IN"=w232, "Error IN"=w234) -> ()  [unwired: 11 in, 2 out]
          }
          event "Snap Next frame": Value Change {
            w248 = T4 0 items=["START_STREAM", "PAUSE_STREAM", "STOP_STREAM"] ("uStreamState IN")
            n159 = event-data() -> ()  [unwired: 1 in, 6 out]
            n160 = property on="Camera Handle" class="DigNum (strict)"() -> ("Value"=w249:u32)  [unwired: 2 in, 2 out]
            n161 = flat-sequence {
              tunnel: w256 -> [w375]
              tunnel: [w375] -> w255
              frame #0 {
                n162 = property on="Waiting for Trigger" class="Bool (strict)"("Value"=TRUE ("Waiting for Trigger")) -> ()  [unwired: 2 in, 2 out]
              }
            }
            n163 = call <vilib>:"MEPU-Acquisition-SetStreamState.vi"("hCamera IN"=w249, "uStreamState IN"=w248, "Error IN"=w255) -> ("hCamera OUT"=w258:u32, "Error OUT"=w257:errorcluster)  [unwired: 11 in]
            n164 = call "Get Buffer Size.vi"("phCamera IN"=w258, "Error IN"=w257) -> ("phCamera OUT"=w262:u32, "uBufferSize OUT"=w260:u32, "uWidth OUT"=w252:u32, "uHeight OUT"=w251:u32, "Error OUT"=w261:errorcluster)  [unwired: 8 in, 1 out]
            n165 = call <vilib>:"MEPU-Acquisition-GetNextFrame.vi"("hCamera IN"=w262, "Mode IN"=enum16{"UseArray", "UsePointer"}."UseArray", "uBufferSize IN"=w260, "Error IN"=w261) -> ("Data OUT"=w254:u8[], "pDescriptor"=w250:T6, "Error OUT"=w253:errorcluster)  [unwired: 7 in, 2 out]
            n166 = property on="Error OUT 2" class="Clust (strict)"("Value"=w253) -> ()  [unwired: 2 in, 2 out]
            n167 = case shown="No Error" w253 {
              tunnel: w254 -> [w266 _]
              tunnel: w252 -> [w265 _]
              tunnel: w251 -> [w264 _]
              tunnel: w250 -> [w263 _]
              frame No Error {
                n168 = property on="Save Data" class="Bool (strict)"() -> ("Value"=w267:bool)  [unwired: 2 in, 2 out]
                n169 = Type Cast(type=u16[] [] ("Data OUT"), x=w266) -> (*(type *) &x=w268:u16[])
                n170 = stacked-sequence {
                  seq-local: [_ _ _ _ w325 _] -> [_ _ _ _ _ w351]
                  seq-local: [_ w277 _ _ _ _] -> [_ _ w311 _ _ _]
                  seq-local: [w272 _ _ _ _ _] -> [_ _ _ _ _ w349]
                  seq-local: [_ _ w301 _ _ _] -> [_ _ _ w316 _ _]
                  tunnel: w268 -> [w276 w286 _ _ _ _]
                  tunnel: w267 -> [_ _ _ _ w324 w350]
                  tunnel: w265 -> [w274 _ _ _ _ _]
                  tunnel: w264 -> [w273 _ _ _ _ _]
                  tunnel: w263 -> [_ w282 _ _ _ _]
                  frame #0 {
                    n171 = Reshape Array(w276, w273, w274) -> (w272:u16[][])
                    n172 = local read "Div"() -> (w271:dbl)
                    n173 = Divide(x=w272, y=w271) -> (x/y=w270:dbl[][])
                    n174 = property on="Waiting for Trigger" class="Bool (strict)"("Value"=FALSE ("Waiting for Trigger")) -> ()  [unwired: 2 in, 2 out]
                    n175 = property on="Focal Spot" class="IntGraph (strict)"("Value"=w270) -> ()  [unwired: 2 in, 2 out]
                    n176 = local write "ROI"(w270) -> ()
                    n177 = local write "Background"(w270) -> ()
                  }
                  frame #1 {
                    n178 = Unbundle By Name(w282) -> ("ROI.fHeight"=w281:dbl, "ROI.fWidth"=w280:dbl)
                    n179 = property on="Background  substraction" class="Bool (strict)"() -> ("Value"=w279:bool)  [unwired: 2 in, 2 out]
                    n180 = To Double Precision Float(number=w286) -> (double precision float=w284:dbl[])
                    n181 = Reshape Array(w284, w281, w280) -> (w285:dbl[][])
                    n182 = Transpose 2D Array(2D array=w285) -> (transposed array=w283:dbl[][])
                    n183 = case shown="False" w279 {
                      tunnel: w283 -> [w294 _]
                      tunnel: [w294 w295] -> w278
                      frame False {
                      }
                      frame True {
                        n184 = control-ref of="ROI"() -> (w297:refnum<vi>)
                        n185 = control-ref of="Background"() -> (w296:refnum<vi>)
                        n186 = call "BackgroundSubstraction.vi"("Background Refnum"=w296, "ROI Refnum"=w297) -> ("Background Sub ROI"=w295:dbl[][])  [unwired: 9 in]
                      }
                    }
                    n187 = for {
                      tunnel: w278 -> [w288] mode=indexing
                      tunnel: [w287] -> w277 mode=indexing
                      n188 = for {
                        tunnel: w288 -> [w290] mode=indexing
                        tunnel: [w289] -> w287 mode=indexing
                        n189 = Less Than 0?(x=w290) -> (x < 0?=w291:bool)
                        n190 = case shown="True" w291 {
                          tunnel: w291 -> [_ _]
                          tunnel: w290 -> [w292 _]
                          tunnel: [w292 0.0] -> w289
                          frame False {
                          }
                          frame True {
                          }
                        }
                      }
                    }
                  }
                  frame #2 {
                    n191 = call "TF_analyse.vi"("image 2D"=w311, "FLUENCE calculation"=TRUE) -> ("FWHM en x"=w307:dbl, "FWHM en y"=w308:dbl, "coupes x & y"=→"?":dbl[][], "intégration totale"=w301:dbl)  [unwired: 19 in, 3 out]
                    n192 = property on="Transmission" class="DigNum (strict)"() -> ("Value"=w298:dbl)  [unwired: 2 in, 2 out]
                    n193 = property on="Duration FWHM (fs)" class="DigNum (strict)"() -> ("Value"=w309:dbl)  [unwired: 2 in, 2 out]
                    n194 = property on="Pulse Energy (mJ)" class="DigNum (strict)"() -> ("Value"=w299:dbl)  [unwired: 2 in, 2 out]
                    n195 = property on="Calibration µm/px" class="DigNum (strict)"() -> ("Value"=w310:dbl)  [unwired: 2 in, 2 out]
                    n196 = Multiply(x=w299, y=w298) -> (x*y=w300:dbl)
                    n197 = call "Calculations.vi"("FWHM x (px)"=w307, "Calibration µm/px"=w310, "Energy in 1 Pulse (mJ)"=w300, "Pulse Duration (fs)"=w309, "FWHM y (px)"=w308) -> ("FWHM y (µm)"=w304:dbl, "FWHM x (µm)"=w305:dbl, "Peak Power (TW)"=w303:dbl, "Integral of Perfect Gaussian (x10^18 W/cm²)"=w302:dbl)  [unwired: 3 in]
                    n198 = property on="Peak power (TW)" class="DigNum (strict)"("Value"=w303) -> ()  [unwired: 2 in, 2 out]
                    n199 = property on="Intensity (gaussian)\nx10^18 W/cm²" class="DigNum (strict)"("Value"=w302) -> ()  [unwired: 2 in, 2 out]
                    n200 = property on="FWHM x (µm)" class="DigNum (strict)"("Value"=w305) -> ()  [unwired: 2 in, 2 out]
                    n201 = property on="FWHM y (µm)" class="DigNum (strict)"("Value"=w304) -> ()  [unwired: 2 in, 2 out]
                  }
                  frame #3 {
                    n202 = property on="Calibration µm/px" class="DigNum (strict)"() -> ("Value"=w317:dbl)  [unwired: 2 in, 2 out]
                    n203 = property on="Duration FWHM (fs)" class="DigNum (strict)"() -> ("Value"=w320:dbl)  [unwired: 2 in, 2 out]
                    n204 = property on="Transmission" class="DigNum (strict)"() -> ("Value"=w322:dbl)  [unwired: 2 in, 2 out]
                    n205 = property on="Pulse Energy (mJ)" class="DigNum (strict)"() -> ("Value"=w323:dbl)  [unwired: 2 in, 2 out]
                    n206 = Compound Arithmetic op=MULTIPLY(w323, w322, 1e-06 ("Transmission")) -> (w315:dbl)
                    n207 = Compound Arithmetic op=MULTIPLY(w320, 1.0645 ("Transmission"), 1e-08 ("Transmission"), w317, w317, w316) -> (w314:dbl)
                    n208 = Divide(x=w315, y=w314) -> (x/y=w313:dbl)
                    n209 = property on="Intensity (measured)\nx10^18 W/cm²" class="DigNum (strict)"("Value"=w313) -> ()  [unwired: 2 in, 2 out]
                  }
                  frame #4 {
                    n210 = case shown="True" w324 {
                      tunnel: [path "" ("File Path") w330] -> w325
                      frame False {
                      }
                      frame True {
                        n211 = property on="Racine chemin de sauvegarde" class="Path"() -> ("Value"=w331:path)  [unwired: 2 in, 2 out]
                        n212 = property on="Nom du fichier" class="Str"() -> ("Value"=w332:string)  [unwired: 2 in, 2 out]
                        n213 = property on="Indice" class="DigNum (strict)"() -> ("Value"=w333:u32)  [unwired: 2 in, 2 out]
                        n214 = property on="Overwrite?" class="Bool (strict)"() -> ("Value"=w334:bool)  [unwired: 2 in, 2 out]
                        n215 = property on="Automatic\nfolder naming" class="Bool (strict)"() -> ("Value"=w327:bool)  [unwired: 2 in, 2 out]
                        n216 = case shown="True" w327 {
                          tunnel: w334 -> [w338 w348]
                          tunnel: w333 -> [w339 w347]
                          tunnel: w332 -> [w340 w346]
                          tunnel: w331 -> [w341 w345]
                          tunnel: [w337 w344] -> w330
                          tunnel: [w336 w343] -> w329
                          tunnel: [w335 w342] -> w328
                          frame False {
                            n217 = call "CheckFolder.vi"("Overwrite?"=w338, "Index"=w339, "File Name"=w340, "Folder Path Control"=w341) -> ("Warning"=w335:bool, "Message"=w336:string, "File Path"=w337:path)  [unwired: 5 in]
                          }
                          frame True {
                            n218 = call "CheckMonthDateFolder.vi"("Overwrite?"=w348, "Index"=w347, "File Name"=w346, "Folder Path Control"=w345) -> ("Warning"=w342:bool, "Message"=w343:string, "File Path"=w344:path)  [unwired: 5 in]
                          }
                        }
                        n219 = property on="Warning" class="Bool (strict)"("Value"=w328) -> ()  [unwired: 2 in, 2 out]
                        n220 = property on="Message" class="Str"("Value"=w329) -> ()  [unwired: 2 in, 2 out]
                      }
                    }
                  }
                  frame #5 {
                    n221 = case shown="True" w350 {
                      tunnel: w351 -> [_ w353]
                      tunnel: w349 -> [_ w352]
                      frame False {
                      }
                      frame True {
                        n222 = Not A Number/Path/Refnum?(number/path/refnum=w353) -> (NaN/Path/Refnum?=w354:bool)
                        n223 = case shown="False" w354 {
                          tunnel: w353 -> [w355 _]
                          tunnel: w352 -> [w360 _]
                          frame False {
                            # "Save Image\nand data"
                            n224 = call "SavePicture.vi"("File Path"=w355, "Image Pixels (U16)"=w360) -> ("error out"=w366:errorcluster)  [unwired: 9 in]
                            n225 = property on="Nom du fichier" class="Str"() -> ("Value"=w356:string)  [unwired: 2 in, 2 out]
                            n226 = property on="Indice" class="DigNum (strict)"() -> ("Value"=w357:u32)  [unwired: 2 in, 2 out]
                            n227 = property on="Exposure Time" class="Slide (strict)"() -> ("Value"=w358:dbl)  [unwired: 2 in, 2 out]
                            n228 = Unbundle By Name(w366) -> ("source"=w363:string, "status"=w364:bool)
                            n229 = call "FindLineAndOverwrite_Double.vi"("Exposure path"=w355, "Name"=w356, "Index"=w357, "Exposure"=w358) -> ("error out"=w359:errorcluster)  [unwired: 11 in]
                            n230 = Unbundle By Name(w359) -> ("status"=w365:bool, "source"=w367:string)
                            n231 = Or(x=w364, y=w365) -> (x .or. y?=w362:bool)
                            n232 = case shown="False" w362 {
                              tunnel: w367 -> [_ w371]
                              tunnel: w363 -> [_ w374]
                              tunnel: "\r\n" -> [_ w372]
                              frame False {
                                n233 = property on="Mode de Sauvegarde" class="Ring (strict)"() -> ("Value"=w369:u16)  [unwired: 2 in, 2 out]
                                n234 = property on="Indice" class="DigNum (strict)"() -> ("Value"=w370:u32)  [unwired: 2 in, 2 out]
                                n235 = Add(x=w370, y=w369) -> (x+y=w368:u32)
                                n236 = property on="Indice" class="DigNum (strict)"("Value"=w368) -> ()  [unwired: 2 in, 2 out]
                              }
                              frame True {
                                n237 = Concatenate Strings(w374, w372, w371) -> (w373:string)
                                n238 = property on="Message" class="Str"("Value"=w373) -> ()  [unwired: 2 in, 2 out]
                              }
                            }
                          }
                          frame True {
                          }
                        }
                      }
                    }
                  }
                }
              }
              frame Error {
              }
            }
          }
          event "Snap current Data": Value Change {
            n239 = event-data() -> ()  [unwired: 1 in, 6 out]
            n240 = stacked-sequence {
              seq-local: [w384 _] -> [_ w400]
              frame #0 {
                n241 = property on="Racine chemin de sauvegarde" class="Path"() -> ("Value"=w380:path)  [unwired: 2 in, 2 out]
                n242 = property on="Nom du fichier" class="Str"() -> ("Value"=w381:string)  [unwired: 2 in, 2 out]
                n243 = property on="Indice" class="DigNum (strict)"() -> ("Value"=w382:u32)  [unwired: 2 in, 2 out]
                n244 = property on="Overwrite?" class="Bool (strict)"() -> ("Value"=w383:bool)  [unwired: 2 in, 2 out]
                n245 = property on="Automatic\nfolder naming" class="Bool (strict)"() -> ("Value"=w377:bool)  [unwired: 2 in, 2 out]
                n246 = case shown="False" w377 {
                  tunnel: [w387 w398] -> w384
                  tunnel: w383 -> [w388 w397]
                  tunnel: w382 -> [w389 w396]
                  tunnel: w381 -> [w390 w395]
                  tunnel: w380 -> [w391 w394]
                  tunnel: [w386 w393] -> w379
                  tunnel: [w385 w392] -> w378
                  frame False {
                    n247 = call "CheckFolder.vi"("Overwrite?"=w388, "Index"=w389, "File Name"=w390, "Folder Path Control"=w391) -> ("Warning"=w385:bool, "Message"=w386:string, "File Path"=w387:path)  [unwired: 5 in]
                  }
                  frame True {
                    n248 = call "CheckMonthDateFolder.vi"("Overwrite?"=w397, "Index"=w396, "File Name"=w395, "Folder Path Control"=w394) -> ("Warning"=w392:bool, "Message"=w393:string, "File Path"=w398:path)  [unwired: 5 in]
                  }
                }
                n249 = property on="Warning" class="Bool (strict)"("Value"=w378) -> ()  [unwired: 2 in, 2 out]
                n250 = property on="Message" class="Str"("Value"=w379) -> ()  [unwired: 2 in, 2 out]
              }
              frame #1 {
                n251 = Not A Number/Path/Refnum?(number/path/refnum=w400) -> (NaN/Path/Refnum?=w399:bool)
                n252 = case shown="False" w399 {
                  tunnel: w400 -> [w404 _]
                  frame False {
                    # "Save Image\nand data"
                    n253 = property on="Focal Spot" class="IntGraph (strict)"() -> ("Value"=w406:dbl[][])  [unwired: 2 in, 2 out]
                    n254 = call "SavePicture.vi"("File Path"=w404, "Image Pixels (U16)"=w406) -> ("error out"=w412:errorcluster)  [unwired: 9 in]
                    n255 = property on="Nom du fichier" class="Str"() -> ("Value"=w403:string)  [unwired: 2 in, 2 out]
                    n256 = property on="Indice" class="DigNum (strict)"() -> ("Value"=w402:u32)  [unwired: 2 in, 2 out]
                    n257 = property on="Exposure Time" class="Slide (strict)"() -> ("Value"=w401:dbl)  [unwired: 2 in, 2 out]
                    n258 = Unbundle By Name(w412) -> ("source"=w409:string, "status"=w410:bool)
                    n259 = call "FindLineAndOverwrite_Double.vi"("Exposure path"=w404, "Name"=w403, "Index"=w402, "Exposure"=w401) -> ("error out"=w405:errorcluster)  [unwired: 11 in]
                    n260 = Unbundle By Name(w405) -> ("status"=w411:bool, "source"=w413:string)
                    n261 = Or(x=w410, y=w411) -> (x .or. y?=w408:bool)
                    n262 = case shown="False" w408 {
                      tunnel: w413 -> [_ w417]
                      tunnel: w409 -> [_ w420]
                      tunnel: "\r\n" -> [_ w418]
                      frame False {
                        n263 = property on="Mode de Sauvegarde" class="Ring (strict)"() -> ("Value"=w415:u16)  [unwired: 2 in, 2 out]
                        n264 = property on="Indice" class="DigNum (strict)"() -> ("Value"=w416:u32)  [unwired: 2 in, 2 out]
                        n265 = Add(x=w416, y=w415) -> (x+y=w414:u32)
                        n266 = property on="Indice" class="DigNum (strict)"("Value"=w414) -> ()  [unwired: 2 in, 2 out]
                      }
                      frame True {
                        n267 = Concatenate Strings(w420, w418, w417) -> (w419:string)
                        n268 = property on="Message" class="Str"("Value"=w419) -> ()  [unwired: 2 in, 2 out]
                      }
                    }
                  }
                  frame True {
                  }
                }
              }
            }
          }
          event "Imager": Value Change {
            n269 = event-data() -> ()  [unwired: 1 in, 6 out]
            n270 = flat-sequence {
              tunnel: [w425] -> w421
              tunnel: w421 -> [w432]
              frame #0 {
                w423 = T4 2 items=["START_STREAM", "PAUSE_STREAM", "STOP_STREAM"] ("uStreamState IN")
                n271 = property on="Camera Handle" class="DigNum (strict)"() -> ("Value"=w422:u32)  [unwired: 2 in, 2 out]
                n272 = call <vilib>:"MEPU-Acquisition-SetStreamState.vi"("hCamera IN"=w422, "uStreamState IN"=w423) -> ("hCamera OUT"=w424:u32)  [unwired: 12 in, 1 out]
                n273 = call <vilib>:"MEPU-Initialization-Uninitialize.vi"("hCamera IN"=w424) -> ()  [unwired: 14 in, 1 out]
              }
              frame #1 {
                n274 = property on="Imager" class="Ring (strict)"() -> ("Strings []"=w430:string[], "RingText.Text"=w429:string, "StringsAndValues[]"=w427:T1)  [unwired: 2 in, 2 out]
                n275 = Search 1D Array(1D array=w430, element=w429) -> (index of element=w428:i32)  [unwired: 1 in]
                n276 = Index Array(array=w427, index=w428) -> (element=w426:cluster{"String":string, "Value":u32})
                n277 = Unbundle By Name(w426) -> ("Value"=w425:u32)
              }
              frame #2 {
                w435 = T2 1 items=["FEATURE_FLAG_PRESENCE                 0x00000001", "FEATURE_FLAG_MANUAL                     0x00000002", "FEATURE_FLAG_AUTO                         0x00000004", "FEATURE_FLAG_ONEPUSH                   0x00000008", "FEATURE_FLAG_OFF                            0x00000010", "FEATURE_FLAG_DESC_SUPPORTED    0x00000020", "FEATURE_FLAG_READ_ONLY               0x00000040"] ("uFlags IN")
                w434 = T3 8 items=["FEATURE_BRIGHTNESS", "FEATURE_EXPOSURE", "FEATURE_SHARPNESS", "FEATURE_WHITE_BAL", "FEATURE_HUE", "FEATURE_SATURATION", "FEATURE_GAMMA", "FEATURE_SHUTTER", "FEATURE_GAIN", "FEATURE_IRIS", "FEATURE_FOCUS", "FEATURE_TEMPERATURE", "FEATURE_TRIGGER", "FEATURE_ZOOM", "FEATURE_PAN", "FEATURE_TILT", "FEATURE_OPT_FILTER", "FEATURE_GPIO", "FEATURE_FRAME_RATE", "FEATURE_ROI", "FEATURE_FLIP", "FEATURE_PIXEL_ADDRESSING", "FEATURE_PIXEL_FORMAT", "FEATURE_EXTENDED_SHUTTER", "FEATURE_AUTO_ROI", "FEATURE_LOOKUP_TABLE", "FEATURE_MEMORY_CHANNEL", "FEATURE_WHITE_SHADING", "FEATURE_ROTATE", "FEATURE_IMAGER_CLK_DIVISOR", "FEATURE_TRIG_WITH_CNTRLD_LIGHT", "FEATURE_MAX_PIXEL_SIZE"] ("uFeatureId IN")
                w441 = T2 1 items=["FEATURE_FLAG_PRESENCE                 0x00000001", "FEATURE_FLAG_MANUAL                     0x00000002", "FEATURE_FLAG_AUTO                         0x00000004", "FEATURE_FLAG_ONEPUSH                   0x00000008", "FEATURE_FLAG_OFF                            0x00000010", "FEATURE_FLAG_DESC_SUPPORTED    0x00000020", "FEATURE_FLAG_READ_ONLY               0x00000040"] ("uFlags IN")
                w442 = T3 22 items=["FEATURE_BRIGHTNESS", "FEATURE_EXPOSURE", "FEATURE_SHARPNESS", "FEATURE_WHITE_BAL", "FEATURE_HUE", "FEATURE_SATURATION", "FEATURE_GAMMA", "FEATURE_SHUTTER", "FEATURE_GAIN", "FEATURE_IRIS", "FEATURE_FOCUS", "FEATURE_TEMPERATURE", "FEATURE_TRIGGER", "FEATURE_ZOOM", "FEATURE_PAN", "FEATURE_TILT", "FEATURE_OPT_FILTER", "FEATURE_GPIO", "FEATURE_FRAME_RATE", "FEATURE_ROI", "FEATURE_FLIP", "FEATURE_PIXEL_ADDRESSING", "FEATURE_PIXEL_FORMAT", "FEATURE_EXTENDED_SHUTTER", "FEATURE_AUTO_ROI", "FEATURE_LOOKUP_TABLE", "FEATURE_MEMORY_CHANNEL", "FEATURE_WHITE_SHADING", "FEATURE_ROTATE", "FEATURE_IMAGER_CLK_DIVISOR", "FEATURE_TRIG_WITH_CNTRLD_LIGHT", "FEATURE_MAX_PIXEL_SIZE"] ("uFeatureId IN")
                n278 = call <vilib>:"MEPU-Initialization-InitializeSystem.vi"() -> ("Error OUT"=w448:errorcluster)  [unwired: 15 in]
                n279 = control-ref of="Exposure Time"() -> (w447:refnum<vi>)
                n280 = call <vilib>:"MEPU-Initialization-Initialize.vi"("uSerialNumber IN"=w432, "Error IN"=w448) -> ("phCamera OUT"=w446:u32, "Error OUT"=w445:errorcluster)  [unwired: 11 in, 1 out]
                n281 = call "Setup Exposure.vi"("Error IN"=w445, "Shutter"=w447, "hCamera IN"=w446) -> ("Error OUT"=w444:errorcluster, "phCamera OUT"=w443:u32)  [unwired: 7 in]
                n282 = Build Array(1.0) -> (w439:dbl[])
                n283 = call <vilib>:"MEPU-CameraFeatures-SetFeature.vi"("hCamera IN"=w443, "uFeatureId IN"=w442, "uFlags IN"=w441, "pParms IN"=w439, "Error IN"=w444) -> ("hCamera OUT"=w433:u32, "Error OUT"=w438:errorcluster)  [unwired: 8 in, 1 out]
                n284 = Build Array(0.0) -> (w436:dbl[])
                n285 = call <vilib>:"MEPU-CameraFeatures-SetFeature.vi"("hCamera IN"=w433, "uFeatureId IN"=w434, "uFlags IN"=w435, "pParms IN"=w436, "Error IN"=w438) -> ("hCamera OUT"=w431:u32)  [unwired: 8 in, 2 out]
                n286 = property on="Camera Handle" class="DigNum (strict)"("Value"=w431) -> ()  [unwired: 2 in, 2 out]
              }
            }
          }
        }
      }
      n287 = property on="Error OUT" class="Clust (strict)"("Value"=w45) -> ()  [unwired: 2 in, 2 out]
    }
    frame #4 {
      w451 = T4 2 items=["START_STREAM", "PAUSE_STREAM", "STOP_STREAM"] ("uStreamState IN")
      # "Ignore errors here to ensure as\ncomplete a clean up as possible."
      n288 = property on="Camera Handle" class="DigNum (strict)"() -> ("Value"=w449:u32)  [unwired: 2 in, 2 out]
      n289 = call <vilib>:"MEPU-Acquisition-SetStreamState.vi"("hCamera IN"=w449, "uStreamState IN"=w451) -> ("hCamera OUT"=w453:u32)  [unwired: 12 in, 1 out]
      n290 = call <vilib>:"MEPU-Initialization-Uninitialize.vi"("hCamera IN"=w453) -> ("Error OUT"=w452:errorcluster)  [unwired: 14 in]
      n291 = stacked-sequence {
        tunnel: w452 -> [_]
        frame #0 {
          n292 = call <vilib>:"MEPU-Initialization-UninitializeSystem.vi"() -> ()  [unwired: 15 in, 1 out]
        }
      }
    }
  }
  n293 = property on="stop" class="Bool (strict)"("Value"=w1) -> ()  [unwired: 2 in, 2 out]
